vi "Control Path.vi"(11 "VerticalSliderControlEditorPanel in":refnum<class "VerticalSliderControlEditorPanel.lvclass">) -> (2 "Control Path":path)   [LabVIEW 2020, in "VolatusGUIControls.lvlib" / "VerticalSliderControlEditorPanel.lvclass"]
uses:
  VerticalSliderControlEditorPanel.lvclass
  VerticalSliderControlEditorPanel.lvclass/VerticalSliderControlEditorPanel.ctl
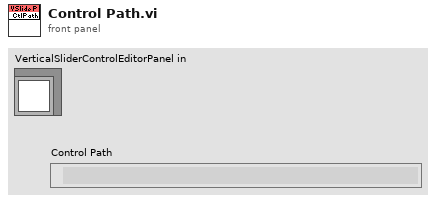
[diagram p1: front panel]
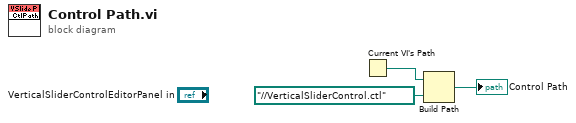
[diagram p0: block diagram]
diagram:
  n1 = Current VI's Path() -> (path=w3:path)
  n2 = Build Path(base path=w3, name or relative path=path "../../VerticalSliderControl.ctl") -> (appended path=→"Control Path":path)
